vi "stimulus control by tracking cycle.vi"(8 "stim enable":bool, 9 "total cycles per stim cycle":u16=10, 10 "lines per stim":u16=42, 11 "line counter":i16) -> (2 "stim on":bool, 3 "use photons":bool)   [LabVIEW 2010]
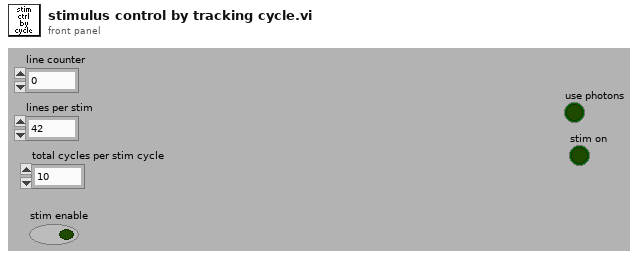
[diagram p1: front panel]
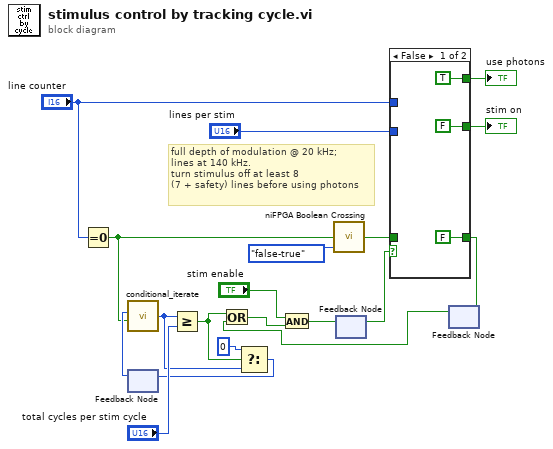
[diagram p0: block diagram]
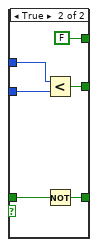
[diagram p2: hidden frame]
diagram:
  # "full depth of modulation @ 20 kHz;\nlines at 140 kHz. \nturn stimulus off at least 8 \n(7 + safety) lines before using photons"
  n1 = Equal To 0?(x="line counter") -> (x = 0?=w8:bool)
  n2 = feedback #1() -> (w16:u16)  [unwired: 1 in]
  n3 = call "conditional_iterate.vi"("iterate?"=w8, "number in"=w16) -> ("number out"=w18:u16)  [unwired: 4 in]
  n4 = Greater Or Equal?(x=w18, y="total cycles per stim cycle") -> (x >= y?=w14:bool)
  n5 = Select(t=u16 0, s=w14, f=w18) -> (s? t:f=w17:u16)
  n6 = feedback-in #1(w17) -> ()
  n7 = call <vilib>:"niFPGA Boolean Crossing.vi"("input"=w8, "direction"=enum8{"either", "false-true", "true-false"}."false-true") -> ("crossing"=w6:bool)  [unwired: 7 in]
  n8 = feedback #2() -> (w5:bool)  [unwired: 1 in]
  n9 = case shown="False" w5 {
    tunnel: "line counter" -> [_ w28]
    tunnel: "lines per stim" -> [_ w27]
    tunnel: [FALSE w26] -> w2
    tunnel: w6 -> [_ w25]
    tunnel: [FALSE w24] -> w4
    tunnel: [TRUE FALSE] -> w1
    frame False {
    }
    frame True {
      n10 = Less?(x=w28, y=w27) -> (x < y?=w26:bool)
      n11 = Not(x=w25) -> (.not. x?=w24:bool)
    }
  }
  "stim on" <- w2
  "use photons" <- w1
  n12 = feedback-in #3(w4) -> ()
  n13 = feedback #3() -> (w3:bool)  [unwired: 1 in]
  n14 = Or(x=w14, y=w3) -> (x .or. y?=w13:bool)
  n15 = And(x="stim enable", y=w13) -> (x .and. y?=w11:bool)
  n16 = feedback-in #2(w11) -> ()
